vi "read_s7_1200 (SubVI).vi"(8 "error in (no error)":errorcluster, 11 "Refnum in":T1) -> (0 "error out":errorcluster, 3 "Refnum out":T1)   [LabVIEW 2024, in "S7-1200_OPCUA.lvlib"]
uses:
  S7-1200_OPCUA.lvlib
  <vilib>/OPCUA/controls/OPC UA Client Refnum.ctl
  <vilib>/OPCUA/controls/NodeIds.ctl
  <vilib>/OPCUA/controls/NodeId.ctl
  <vilib>/OPCUA/client/Multiple Read Bool.vi
  <vilib>/OPCUA/client/Multiple Read UInt16.vi
  <vilib>/OPCUA/NI OPC UA Client.lvlib
  <vilib>/platform/TimedLoop/XDataNode/XDataNode.xnode
  <vilib>/Platform/TimedLoop/XDataNode/nitl_modes.ctl
  <vilib>/Platform/TimedLoop/XDataNode/XDNodeRunTimeDep.lvlib
  <vilib>/Platform/TimedLoop/XDataNode/wakeup.ctl
  <vilib>/Platform/TimedLoop/XDataNode/timing_clust.ctl
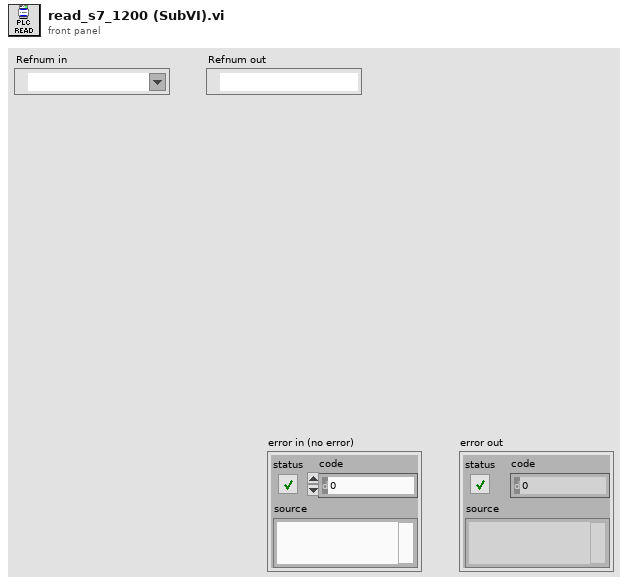
[diagram p1: front panel]
types:
  T1 = typedef "OPC UA Client Refnum.ctl" = refnum<k21>
  T2 = typedef "XDNodeRunTimeDep.lvlib/timing_clust.ctl" = cluster{"Expected End [f-1]":u64, "Actual End [f-1]":u64, "Finished Late? [f-1]":bool, "Expected End [i-1]":u64, "Actual End [i-1]":u64, "Finished Late? [i-1]":bool, "Expected Start [i]":u64, "Actual Start [i]":u64, "Expected Start [f]":u64, "Actual Start [f]":u64, "Source Name":string, "Structure Name":string, "Period":i64, "Deadline":i64, "Offset":i64, "Start":i64, "Priority":i32, "Timeout":i32, "Mode":T3, "Wakeup Reason":T4, "Error":errorcluster, "Source Type":string, "Secondary Source Type":string, "Global End Time":u64, "Global Start Time":u64, "Frame Duration":u64, "Iteration Duration":u64, "Assigned CPU":i32, "I/O Scan Engine Mode":u32}
  T3 = typedef "XDNodeRunTimeDep.lvlib/nitl_modes.ctl" = enum32{"No Change", "Process missed periods, maintain original phase", "Discard missed periods, maintain original phase", "Process missed periods, ignore original phase", "Discard missed periods, ignore original phase"}
  T4 = typedef "XDNodeRunTimeDep.lvlib/wakeup.ctl" = enum32{"Normal", "Aborted", "Asynchronous wakeup", "Timing source error", "Timed loop error", "Timeout"}
  T5 = typedef "NodeIds.ctl" = T6[]
  T6 = typedef "NodeId.ctl" = string
  T7 = typedef "OPC UA StatusCode.ctl" = u32
  T8 = cluster{"node ID":T6, "value ":bool, "timestamp":timestamp, "status":T7}[]
  T9 = cluster{"node ID":T6, "value ":u16, "timestamp":timestamp, "status":T7}[]
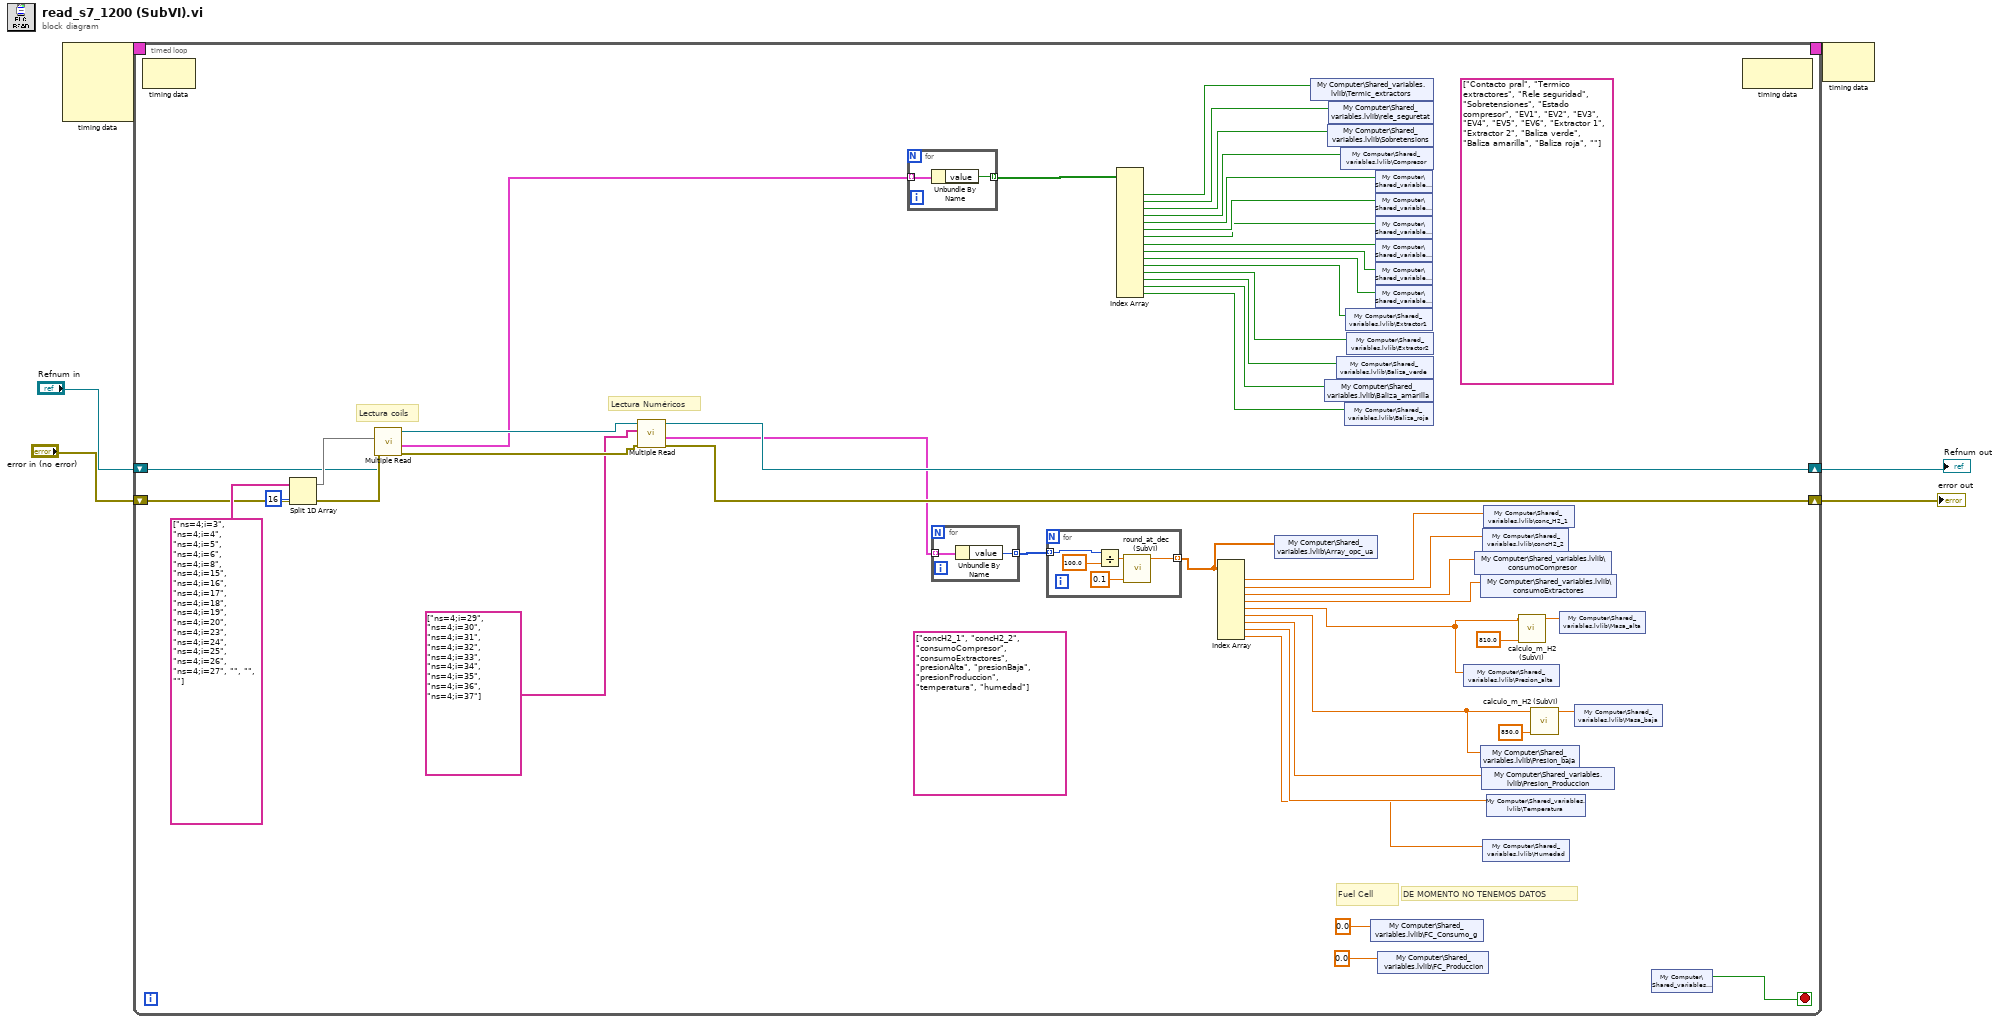
[diagram p0: block diagram]
diagram:
  n1 = node-c288() -> (w2:T2)  [unwired: 4 in]
  n2 = timed-loop {
    timing: w2 -> [_]
    timing-out: [_] -> w1
    shift-right: [w52] -> w6
    shift-left: "error in (no error)" -> [w45]
    shift-right: [w50] -> w5
    shift-left: "Refnum in" -> [w44]
    stop <- w7 stop-if-true
    (unwired) string[] ["concH2_1", "concH2_2", "consumoCompresor", "consumoExtractores", "presionAlta", "presionBaja", "presionProduccion", "temperatura", "humedad"] ("Key Array")
    (unwired) string[] ["Contacto pral", "Termico extractores", "Rele seguridad", "Sobretensiones", "Estado compresor", "EV1", "EV2", "EV3", "EV4", "EV5", "EV6", "Extractor 1", "Extractor 2", "Baliza verde", "Baliza amarilla", "Baliza roja", ""]
    # "DE MOMENTO NO TENEMOS DATOS"
    # "Fuel Cell"
    # "Lectura Numéricos"
    # "Lectura coils"
    n3 = node-c288() -> ()  [unwired: 1 in, 1 out]
    n4 = Split 1D Array(array=T5 ["ns=4;i=3", "ns=4;i=4", "ns=4;i=5", "ns=4;i=6", "ns=4;i=8", "ns=4;i=15", "ns=4;i=16", "ns=4;i=17", "ns=4;i=18", "ns=4;i=19", "ns=4;i=20", "ns=4;i=23", "ns=4;i=24", "ns=4;i=25", "ns=4;i=26", "ns=4;i=27", "", "", ""] ("node IDs"), index=16) -> (first subarray=w47:T5)  [unwired: 1 out]
    n5 = call-poly <vilib>:"Multiple Read.vi"("error in (no error)"=w45, "node IDs"=w47, "OPC UA client refnum in"=w44) -> ("error out"=w51:errorcluster, "results"=w43:T8, "OPC UA client refnum out"=w49:T1)  [unwired: 5 in, 1 out]
    n6 = call-poly <vilib>:"Multiple Read.vi"("error in (no error)"=w51, "node IDs"=T5 ["ns=4;i=29", "ns=4;i=30", "ns=4;i=31", "ns=4;i=32", "ns=4;i=33", "ns=4;i=34", "ns=4;i=35", "ns=4;i=36", "ns=4;i=37"], "OPC UA client refnum in"=w49) -> ("error out"=w52:errorcluster, "results"=w26:T9, "OPC UA client refnum out"=w50:T1)  [unwired: 5 in, 1 out]
    n7 = for {
      tunnel: w43 -> [w61] mode=indexing
      tunnel: [w60] -> w42 mode=indexing
      n8 = Unbundle By Name(w61) -> ("value"=w60:bool)
    }
    n9 = for {
      tunnel: w26 -> [w59] mode=indexing
      tunnel: [w58] -> w20 mode=indexing
      n10 = Unbundle By Name(w59) -> ("value"=w58:u16)
    }
    n11 = for {
      tunnel: w20 -> [w54] mode=indexing
      tunnel: [w53] -> w15 mode=indexing
      n12 = Divide(x=w54, y=100.0) -> (x/y=w55:dbl)
      n13 = call "round_at_dec (SubVI).vi"("Decimal"=0.1, "numeric in"=w55) -> ("Numeric out"=w53:dbl)  [unwired: 9 in]
    }
    n14 = Index Array(array=w42) -> (element #2=w41:bool, element #3=w40:bool, element #4=w39:bool, element #5=w38:bool, element #6=w37:bool, element #7=w36:bool, element #8=w35:bool, element #9=w34:bool, element #10=w33:bool, element #11=w32:bool, element #12=w9:bool, element #13=w8:bool, element #14=w31:bool, element #15=w30:bool, element #16=w29:bool)  [unwired: 16 in, 1 out]
    n15 = Index Array(array=w15) -> (element #1=w10:dbl, element #2=w11:dbl, element #3=w12:dbl, element #4=w13:dbl, element #5=w19:dbl, element #6=w18:dbl, element #7=w14:dbl, element #8=w17:dbl, element #9=w16:dbl)  [unwired: 9 in]
    n16 = shared-variable "My Computer\\Shared_variables.lvlib\\Array_opc_ua"(w15) -> ()  [unwired: 1 in, 1 out]
    n17 = shared-variable "My Computer\\Shared_variables.lvlib\\Termic_extractors"(w41) -> ()  [unwired: 1 in, 1 out]
    n18 = shared-variable "My Computer\\Shared_variables.lvlib\\Baliza_amarilla"(w30) -> ()  [unwired: 1 in, 1 out]
    n19 = shared-variable "My Computer\\Shared_variables.lvlib\\Sobretensions"(w39) -> ()  [unwired: 1 in, 1 out]
    n20 = shared-variable "My Computer\\Shared_variables.lvlib\\rele_seguretat"(w40) -> ()  [unwired: 1 in, 1 out]
    n21 = shared-variable "My Computer\\Shared_variables.lvlib\\Baliza_verde"(w31) -> ()  [unwired: 1 in, 1 out]
    n22 = shared-variable "My Computer\\Shared_variables.lvlib\\Compresor"(w38) -> ()  [unwired: 1 in, 1 out]
    n23 = shared-variable "My Computer\\Shared_variables.lvlib\\Baliza_roja"(w29) -> ()  [unwired: 1 in, 1 out]
    n24 = shared-variable "My Computer\\Shared_variables.lvlib\\Extractor1"(w9) -> ()  [unwired: 1 in, 1 out]
    n25 = shared-variable "My Computer\\Shared_variables.lvlib\\Extractor2"(w8) -> ()  [unwired: 1 in, 1 out]
    n26 = shared-variable "My Computer\\Shared_variables.lvlib\\FC_Consumo_g"(0.0 ("g H2 consumidos por la FC")) -> ()  [unwired: 1 in, 1 out]
    n27 = shared-variable "My Computer\\Shared_variables.lvlib\\EV1"(w37) -> ()  [unwired: 1 in, 1 out]
    n28 = shared-variable "My Computer\\Shared_variables.lvlib\\EV2"(w36) -> ()  [unwired: 1 in, 1 out]
    n29 = shared-variable "My Computer\\Shared_variables.lvlib\\EV3"(w35) -> ()  [unwired: 1 in, 1 out]
    n30 = shared-variable "My Computer\\Shared_variables.lvlib\\EV4"(w34) -> ()  [unwired: 1 in, 1 out]
    n31 = shared-variable "My Computer\\Shared_variables.lvlib\\EV5"(w33) -> ()  [unwired: 1 in, 1 out]
    n32 = shared-variable "My Computer\\Shared_variables.lvlib\\EV6"(w32) -> ()  [unwired: 1 in, 1 out]
    n33 = shared-variable "My Computer\\Shared_variables.lvlib\\FC_Produccion"(0.0 ("Producción FC")) -> ()  [unwired: 1 in, 1 out]
    n34 = shared-variable "My Computer\\Shared_variables.lvlib\\Presion_alta"(w19) -> ()  [unwired: 1 in, 1 out]
    n35 = shared-variable "My Computer\\Shared_variables.lvlib\\consumoCompresor"(w12) -> ()  [unwired: 1 in, 1 out]
    n36 = shared-variable "My Computer\\Shared_variables.lvlib\\consumoExtractores"(w13) -> ()  [unwired: 1 in, 1 out]
    n37 = shared-variable "My Computer\\Shared_variables.lvlib\\Presion_baja"(w18) -> ()  [unwired: 1 in, 1 out]
    n38 = shared-variable "My Computer\\Shared_variables.lvlib\\Presion_Produccion"(w14) -> ()  [unwired: 1 in, 1 out]
    n39 = shared-variable "My Computer\\Shared_variables.lvlib\\concH2_2"(w11) -> ()  [unwired: 1 in, 1 out]
    n40 = shared-variable "My Computer\\Shared_variables.lvlib\\Humedad"(w16) -> ()  [unwired: 1 in, 1 out]
    n41 = shared-variable "My Computer\\Shared_variables.lvlib\\conc_H2_1"(w10) -> ()  [unwired: 1 in, 1 out]
    n42 = shared-variable "My Computer\\Shared_variables.lvlib\\Temperatura"(w17) -> ()  [unwired: 1 in, 1 out]
    n43 = call "calculo_m_H2 (SubVI).vi"("V"=810.0, "P"=w19) -> ("Numeric out"=w24:dbl)  [unwired: 9 in]
    n44 = call "calculo_m_H2 (SubVI).vi"("V"=850.0, "P"=w18) -> ("Numeric out"=w22:dbl)  [unwired: 9 in]
    n45 = shared-variable "My Computer\\Shared_variables.lvlib\\Masa_alta"(w24) -> ()  [unwired: 1 in, 1 out]
    n46 = shared-variable "My Computer\\Shared_variables.lvlib\\Masa_baja"(w22) -> ()  [unwired: 1 in, 1 out]
    n47 = shared-variable "My Computer\\Shared_variables.lvlib\\Stop"() -> (w7:bool)  [unwired: 1 in, 1 out]
    n48 = node-c288() -> ()  [unwired: 1 in, 1 out]
  }
  "error out" <- w6
  "Refnum out" <- w5
  n49 = node-c288(w1) -> ()  [unwired: 1 out]
